vi "Write DAQ FIFO.vi"(6 "FIFO Timestamps":T2, 8 "error in (no error)":errorcluster, 9 "Timeout (ms)":i32, 10 "Data In":T1[](array[typedef]), 11 "CIF_NIChn_FIFO_DAQ in":refnum<class "CIF_NIChn_FIFO_DAQ_DVR.lvclass">) -> (0 "error out":errorcluster, 1 "timed out?":bool, 2 "Data Out":T1[](array[typedef]), 3 "CIF_NIChn_FIFO_DAQ out":refnum<class "CIF_NIChn_FIFO_DAQ_DVR.lvclass">)   [LabVIEW 2021, in "CIF_NIChn_FIFO_DAQ_DVR.lvclass"]
uses:
  CIF_NIChn_FIFO_DAQ_DVR.lvclass
  D:/dev/Packages/Channel_Manager/src/CIFChannels/CIFChannels.lvclass
  D:/dev/Packages/Channel_Manager/src/CIF_NIChn/FIFO_U8/CIF_NIChn_Fifo_U8.lvclass
  ChannelCommon/typedef/TimeStamps.ctl
  ChannelCommon/typedef/Datatype Waveform.ctl
  CIFChannels/CIFChannels.lvclass/CIFChannels.ctl
  CIF_NIChn_FIFO_DAQ_DVR.lvclass/CIF_NIChn_FIFO_DAQ_DVR.ctl
  FIFO_U8/CIF_NIChn_Fifo_U8.lvclass/CIF_NIChn_Fifo_U8.ctl
  <vilib>/CIF Foundation/CIF Utilities/Statistics/I64/Stats_I64_CIF_U.lvclass/Stats_I64_CIF_U.ctl
  NIChn/CIF_NIChn.lvclass/CIF_NIChn.ctl
  FIFO_U8/Accessors/Read Payload.vi
  NIChn/Accessors/Read CIF Channel.vi
  CIFChannels/Utilities/Update Channel Benchmark.vi
  FIFO_U8/SubVIs/Core Write U8 FIFO.vi/1bad10da-a98b-49ee-b03a-18b497e396df.vi
  FIFO_U8/SubVIs/Core Write U8 FIFO.vi/70f860b1-5d4a-43dc-b0c2-c9446e8447f7.vi
  <vilib>/CIF Foundation/CIF Channels/CIFChannels/Top Level/Write U8 Array.vi
  CIFChannels/Accessors/Read FIFO Header.vi
  SubVIs/DVR Flatten.vi
  FIFO_U8/Accessors/Write Payload.vi
  SubVIs/Get Waveform DVRs.vi
  CIFChannels/Utilities/Update Flatten Benchmark.vi
  SubVIs/Flatten.vi/587a020d-d764-4ff7-9451-6b801beca2fa.vi
  SubVIs/Flatten.vi/b511efe2-f594-4971-95dc-73ac55586360.vi
  CIFChannels/Accessors/Read FIFO Retry on Timeout.vi
  <vilib>/CIF Foundation/CIF Utilities/Statistics/I64/X1 minus X0.vi
  <vilib>/CIF Foundation/CIF Utilities/Time/System Time/Get System Time.vi
  <vilib>/CIF Foundation/CIF Channels/CIFChannels/SubVIs/Get dll Path.vi
  <vilib>/CIF Foundation/CIF Channels/CIFChannels/SubVIs/Get Requested Size.vi
  <vilib>/CIF Foundation/CIF Utilities/DataTypes/Flatten U64.vi
  CIFChannels/Utilities/Create Flattened FIFO Header.vi
  <vilib>/CIF Foundation/CIF Utilities/Statistics/I64/X1 minus X0.vi/dfabcf33-0dbc-4041-80a5-3dc0c86d2989.vi
  <vilib>/CIF Foundation/CIF Utilities/Time/System Time/LabVIEW Time to TAI Time.vi
  ChannelCommon/Utilities/Flatten Header.vi
  CIFChannels/Utilities/Update FIFO Header.vi
  <vilib>/CIF Foundation/CIF Utilities/Statistics/I64/X1 minus X0.vi/dfabcf33-0dbc-4041-80a5-3dc0c86d2989.vi/9eb60a9a-770f-4d2d-8b3f-8465c267ecc9.vi
  <vilib>/CIF Foundation/CIF Utilities/DataTypes/Flatten I64.vi
  FIFO_U8/CIF_NIChn_Fifo_U8.lvclass
  D:/dev/Packages/Channel_Manager/src/CIF_NIChn/NIChn/CIF_NIChn.lvclass
  ChannelCommon/ChannelCommon.lvlib
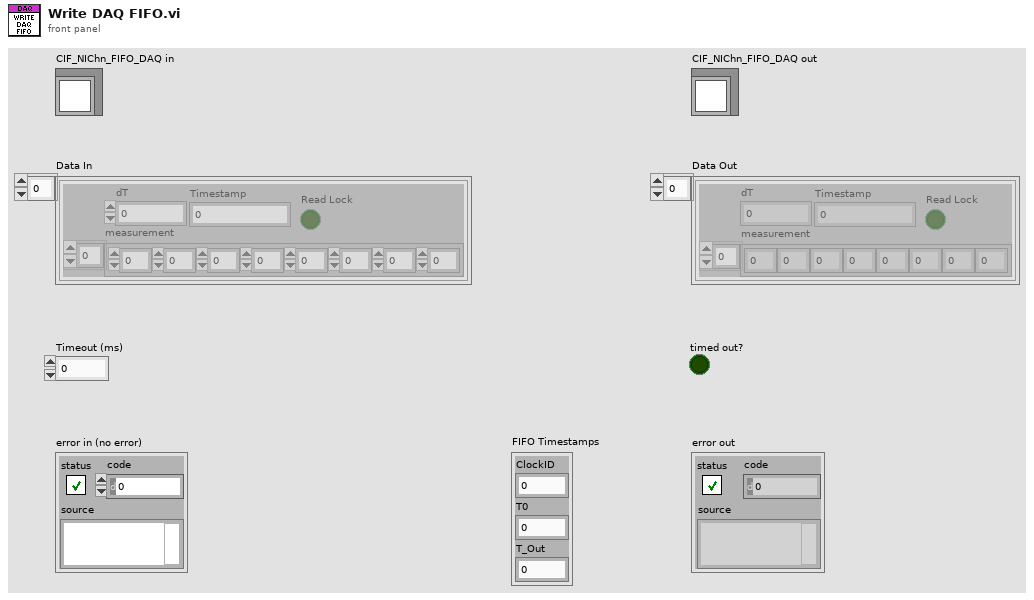
[diagram p1: front panel]
types:
  T1 = typedef "ChannelCommon.lvlib/Datatype Waveform.ctl" = cluster{"measurement":dbl[], "dT":dbl, "Timestamp":i64, "Read Lock":bool}
  T2 = typedef "ChannelCommon.lvlib/TimeStamps.ctl" = cluster{"ClockID":u8, "T0":i64, "T_Out":i64}
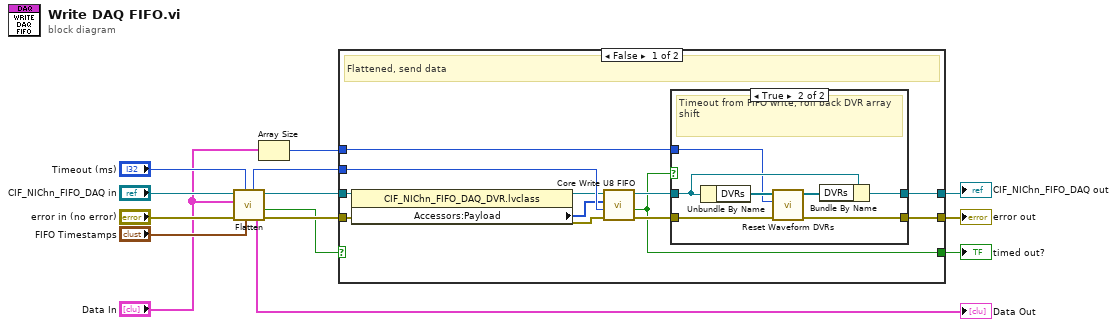
[diagram p0: block diagram]
diagram:
  n1 = call "Flatten.vi"("FIFO Timestamps"="FIFO Timestamps", "Timeout (ms)"="Timeout (ms)", "error in (no error)"="error in (no error)", "Data In"="Data In", "CIF_NIChn_FIFO_DAQ in"="CIF_NIChn_FIFO_DAQ in") -> ("error out"=w4:errorcluster, "timed out?"=w3:bool, "Data Out"=→"Data Out":T1[], "CIF_NIChn_FIFO_DAQ out"=w5:refnum<class "CIF_NIChn_FIFO_DAQ_DVR.lvclass">, "Remaining timeout (ms)"=w6:i32)  [unwired: 2 in]
  n2 = Array Size(array="Data In") -> (size(s)=w14:i32)
  n3 = case shown="False" w3 {
    selector: w3 -> [_ w36]
    tunnel: w4 -> [w18 w37]
    tunnel: w5 -> [w19 w38]
    tunnel: [w26 w38] -> w12
    tunnel: [w20 w36] -> w13
    tunnel: [w25 w37] -> w11
    tunnel: w6 -> [w23 _]
    tunnel: w14 -> [w24 _]
    frame False {
      # "Flattened, send data"
      n4 = property class="CIF_NIChn_FIFO_DAQ_DVR.lvclass"(reference=w19, error in=w18) -> (reference out=w17:refnum<class "CIF_NIChn_FIFO_DAQ_DVR.lvclass">, error out=w15:errorcluster, "Accessors:Payload"=w16:u8[])
      n5 = call "Core Write U8 FIFO.vi"("error in (no error)"=w15, "Timeout (ms)"=w23, "U8 With Header"=w16, "CIFFIFO in"=w17) -> ("error out"=w22:errorcluster, "timed out?"=w20:bool, "CIFFIFO out"=w21:refnum<class "CIF_NIChn_FIFO_DAQ_DVR.lvclass">)  [unwired: 5 in]
      n6 = case shown="True" w20 {
        tunnel: w21 -> [w28 w35]
        tunnel: [w28 w34] -> w26
        tunnel: w22 -> [w27 w33]
        tunnel: [w27 w32] -> w25
        tunnel: w24 -> [_ w29]
        frame False {
        }
        frame True {
          # "Timeout from FIFO write, roll back DVR array shift"
          n7 = Unbundle By Name(w35) -> ("DVRs"=w30:refnum<data-value>[])
          n8 = call "Reset Waveform DVRs.vi"("error in (no error)"=w33, "Number of Waveforms"=w29, "DVR Circular Buffer in"=w30) -> ("error out"=w32:errorcluster, "DVR Circular Buffer out"=w31:refnum<data-value>[])  [unwired: 7 in]
          n9 = Bundle By Name(cluster=w35, "DVRs"=w31) -> (w34:refnum<class "CIF_NIChn_FIFO_DAQ_DVR.lvclass">)
        }
      }
    }
    frame True {
      # "Timeout getting unlocked DVRs"
    }
  }
  "error out" <- w11
  "CIF_NIChn_FIFO_DAQ out" <- w12
  "timed out?" <- w13
